vi "Get Database Information.vi"() -> ()   [LabVIEW 2023]
doc: "This example returns information contained in a database named LabVIEW.mdb located in the LabVIEW examples>>database directory. The information consists of the table names, column names, data types, and data sizes."
uses:
  <vilib>/addons/database/Connection.llb/DB Tools Open Connec (Path).vi
  <vilib>/addons/database/NI_Database_API.lvlib
panel:
  out "Database Information":string[][](table)
  # "Overview: Demonstrates how to retrieve information on all tables in a database.\nRequirements: Database Connectivity Toolkit\nInstructions:\nRun the VI. Information about all tables in the LabVIEW.mdb database is displayed."
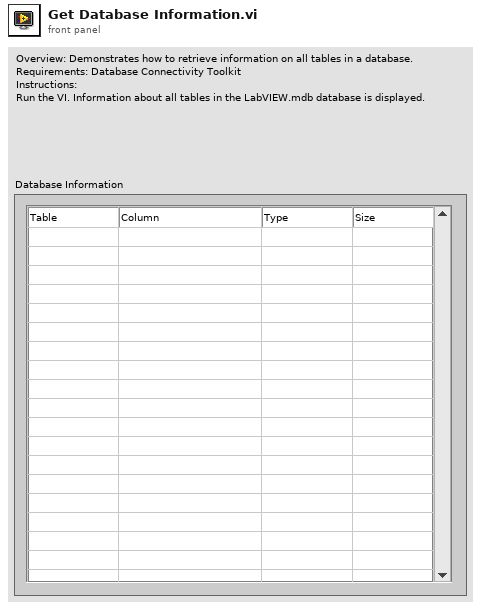
[diagram p1: front panel]
types:
  T1 = typedef "NI_Database_API.lvlib/Conn ObjectReference.ctl" = refnum<k1>
  T2 = typedef "NI_Database_API.lvlib/DB Tools DataTypes.ctl" = enum16{"String", "Long (I32)", "Single (SGL)", "Double (DBL)", "Date/Time", "Binary"}
  T3 = cluster{"name":string, "database data type":T2, "defined size":i32}[]
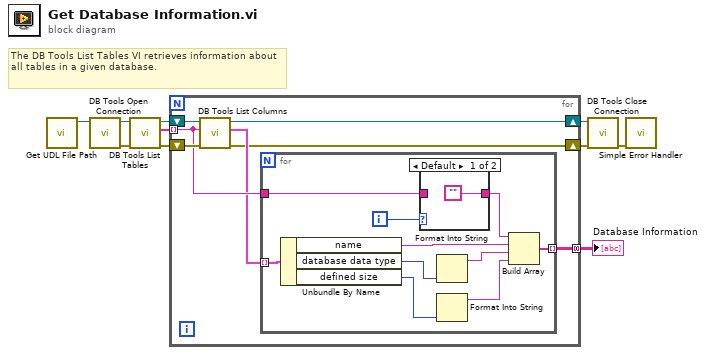
[diagram p0: block diagram]
diagram:
  # "The DB Tools List Tables VI retrieves information about all tables in a given database."
  n1 = call "Get UDL File Path.vi"() -> ("UDL file path"=w2:path)  [unwired: 11 in]
  n2 = call-poly <vilib>:"DB Tools Open Connection.vi"("connection information"=w2) -> ("error out"=w10:errorcluster, "connection reference"=w9:T1)  [unwired: 7 in]
  n3 = call <vilib>:"DB Tools List Tables.vi"("error in (no error)"=w10, "connection reference"=w9) -> ("error out"=w7:errorcluster, "tables"=w6:string[], "connection reference out"=w8:T1)  [unwired: 3 in]
  n4 = for {
    shift-right: [w13] -> w5
    shift-left: w7 -> [w17]
    tunnel: w6 -> [w15] mode=indexing
    shift-right: [w12] -> w4
    shift-left: w8 -> [w16]
    tunnel: [w11] -> w1 mode=concatenating
    n5 = call <vilib>:"DB Tools List Columns.vi"("error in (no error)"=w17, "table"=w15, "connection reference"=w16) -> ("error out"=w13:errorcluster, "column information"=w14:T3, "connection reference out"=w12:T1)  [unwired: 1 in, 1 out]
    n6 = for {
      tunnel: w15 -> [w26]
      tunnel: w14 -> [w23] mode=indexing
      tunnel: [w25] -> w11 mode=indexing
      i -> [w27]
      n7 = Unbundle By Name(w23) -> ("name"=w22:string, "database data type"=w21:T2, "defined size"=w19:i32)
      n8 = case shown="Default" w27 {
        tunnel: w26 -> [_ w29]
        tunnel: ["" w29] -> w24
        frame Default {
        }
        frame 0 {
        }
      }
      n9 = Format Into String(w21) -> (resulting string=w20:string)  [unwired: 3 in, 1 out]
      n10 = Format Into String(w19) -> (resulting string=w18:string)  [unwired: 3 in, 1 out]
      n11 = Build Array(w24, w22, w20, w18) -> (w25:string[])
    }
  }
  "Database Information" <- w1
  n12 = call <vilib>:"DB Tools Close Connection.vi"("error in (no error)"=w5, "connection reference"=w4) -> ("error out"=w3:errorcluster)  [unwired: 5 in]
  n13 = call <vilib>:"Simple Error Handler.vi"("error in (no error)"=w3) -> ()  [unwired: 4 in, 5 out]
